vi "forwardByNavX_theSide(queuesWithNavX).vi"(8 "error in (no error)":errorcluster, 11 "distance the side":u32) -> (0 "error out":errorcluster)   [LabVIEW 2017]
uses:
  <vilib>/myRIO/Common/Instrument Driver Framework/Utilities/typedefs/FPGA Ref Manager Action Enum.ctl
  <vilib>/myRIO/Instrument Drivers/Onboard IO/I2C/typedefs/I2C Reference.ctl
  <vilib>/myRIO/Common/Instrument Driver Framework/Utilities/typedefs/myRIO Generic Hardware Reference.ctl
  <vilib>/myRIO/Common/Instrument Driver Framework/Utilities/typedefs/Hardware Version Enum.ctl
  <vilib>/myRIO/Common/Instrument Driver Framework/Utilities/typedefs/myRIO v1.0 Reference.ctl
  <vilib>/myRIO/Common/Instrument Driver Framework/Utilities/typedefs/Generic FPGA Reference.ctl
  <vilib>/myRIO/Common/Instrument Driver Framework/myRIO v1.0/I2C/typedefs/I2C Channels Enum.ctl
  <vilib>/myRIO/Instrument Drivers/Onboard IO/I2C/typedefs/I2C Configuration.ctl
  <vilib>/myRIO/Instrument Drivers/Onboard IO/I2C/typedefs/I2C Transfer Rate.ctl
  <vilib>/userdefined/High Color/nirio_resource_hc.ctl
  <vilib>/myRIO/Common/Instrument Driver Framework/myRIO v1.0/I2C/vis/myRIO v1.1 Open I2C.vi
  <vilib>/myRIO/Common/Instrument Driver Framework/Utilities/vis/Validate Channels.vi
  <vilib>/myRIO/Common/Instrument Driver Framework/myRIO v1.0/I2C/vis/myRIO v1.0 Reserve I2C.vi
  <vilib>/myRIO/Common/Instrument Driver Framework/myRIO v1.0/I2C/vis/myRIO v1.0 Close I2C.vi
  <vilib>/myRIO/Common/Instrument Driver Framework/myRIO v1.0/I2C/vis/myRIO v1.0 Build MUX Configuration I2C.vi
  <vilib>/myRIO/Common/Instrument Driver Framework/myRIO v1.0/Resource Manager/vis/myRIO v1.0 Reserve Channel List.vi
  <vilib>/myRIO/Common/Instrument Driver Framework/myRIO v1.0/I2C/vis/myRIO v1.0 Unreserve I2C.vi
  <vilib>/myRIO/Common/Instrument Driver Framework/myRIO v1.0/Resource Manager/vis/myRIO v1.0 Create Configuration List.vi
  <vilib>/myRIO/Common/Instrument Driver Framework/myRIO v1.0/Resource Manager/vis/myRIO v1.0 Reserve Channel.vi
  <vilib>/myRIO/Common/Instrument Driver Framework/myRIO v1.0/Resource Manager/vis/myRIO v1.0 Unreserve Channel.vi
  <vilib>/myRIO/Common/Instrument Driver Framework/myRIO v1.0/Resource Manager/vis/myRIO v1.0 Unreserve Channel List.vi
  <vilib>/myRIO/Common/Instrument Driver Framework/myRIO v1.0/Resource Manager/vis/myRIO v1.0 Build Mutex Name.vi
  <vilib>/Utility/VariantDataType/GetNumericInfo.vi
  <vilib>/Utility/error.llb/Error Cluster From Error Code.vi
  <vilib>/myRIO/Common/Instrument Driver Framework/myRIO v1.0/myRIO v1.1 Open.vi
  <vilib>/myRIO/Common/Instrument Driver Framework/Utilities/vis/IO Manager.vi
  <vilib>/myRIO/Common/Instrument Driver Framework/Utilities/vis/Configuration Manager.vi
  <vilib>/myRIO/Common/Instrument Driver Framework/myRIO v1.0/Resource Manager/vis/myRIO v1.0 Configure IO.vi
  <vilib>/myRIO/Common/Instrument Driver Framework/myRIO v1.0/myRIO v1.0 Close.vi
  <vilib>/Instr/_visa.llb/VISA Configure Serial Port (Instr).vi
  <vilib>/myRIO/Common/Instrument Driver Framework/myRIO v1.0/I2C/vis/myRIO v1.0 Shutdown I2C.vi
  <vilib>/myRIO/Instrument Drivers/Onboard IO/I2C/vis/myRIO I2C Open.xnode
  <vilib>/myRIO/Instrument Drivers/Onboard IO/I2C/I2C.lvlib
panel:
  out "axis Z(paste)":ext
  out "main angle":ext
  out "right":dbl
  out "left":dbl
  out "zero angle":ext
  in  "Stop Button":bool
  out "axis Z(after)":ext
  # "--- отклонения от нулевого угла"
  # "PWM"
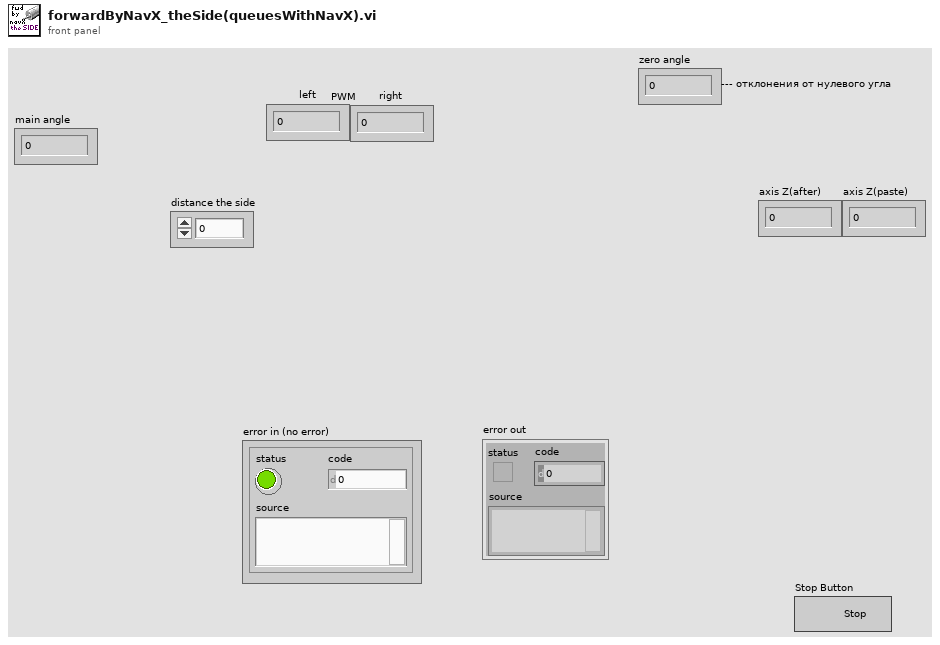
[diagram p1: front panel]
types:
  T1 = typedef "FPGA Ref Manager Action Enum.ctl" = enum16{"Get", "Set", "Reset"}
  T2 = typedef "I2C.lvlib/I2C Reference.ctl" = cluster{"myRIO Reference":T3, "I2C Channels Enum":T7, "I2C Configuration":T8}
  T3 = typedef "myRIO Generic Hardware Reference.ctl" = cluster{"myRIO Model":T4, "myRIO Hardware Reference":T5}
  T4 = typedef "Hardware Version Enum.ctl" = enum16{"Unknown", "myRIO-1900", "myRIO-1950", "roboRIO", "NI ELVIS RIO CM"}
  T5 = typedef "myRIO v1.0 Reference.ctl" = cluster{"Generic FPGA Reference":T6, "Allow multiple opens":bool}
  T6 = typedef "Generic FPGA Reference.ctl" = refnum<k20>
  T7 = typedef "I2C Channels Enum.ctl" = enum16{"Not Connected", "A/I2C", "B/I2C", "I2C/I2C"}
  T8 = typedef "I2C.lvlib/I2C Configuration.ctl" = cluster{"I2C Transfer Rate":T9}
  T9 = typedef "I2C.lvlib/I2C Transfer Rate.ctl" = enum16{"Standard mode (100 kbps)", "Fast mode (400 kbps)"}
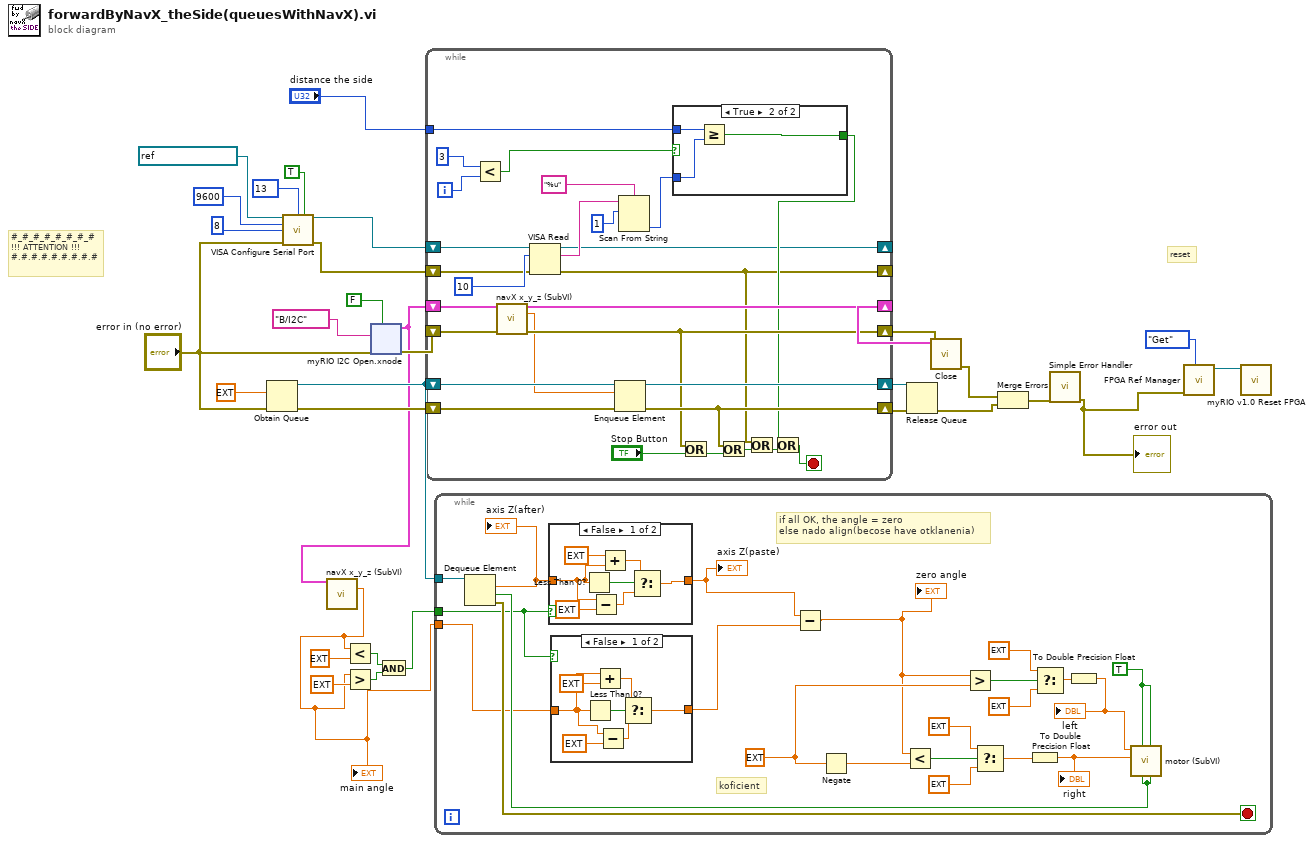
[diagram p0: block diagram]
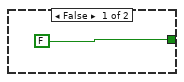
[diagram p4: hidden frame]
diagram:
  # "#_#_#_#_#_#_#_#\n!!! ATTENTION !!!\n#.#.#.#.#.#.#.#.#"
  # "reset"
  n1 = Obtain Queue(element data type=ext 0.0 ("value Z"), error in (no error)="error in (no error)") -> (queue out=w20:refnum<queue>, error out=w32:errorcluster)  [unwired: 3 in, 1 out]
  n2 = call-poly "VISA Configure Serial Port"("VISA resource name"=refnum<visa-resource-name> "ASRL2::INSTR" ("UART selector"), "termination char\n(0xA = '\\n' = LF)"=u8 13 ("termination char = CR"), "Enable Termination\nChar (T)"=TRUE ("enable termination char"), "baud rate (9600)"=u32 9600 ("baud rate"), "data bits (8)"=u16 8 ("data bits"), "error in (no error)"="error in (no error)") -> ("VISA resource name out"=w2:refnum<visa-resource-name>, "error out"=w3:errorcluster)  [unwired: 8 in]
  n3 = xnode "myRIO I2C Open.xnode"("error in (no error)"="error in (no error)", "Allow multiple opens?"=FALSE, "Channel Name"=tag "B/I2C") -> ("error out"=w25:errorcluster, "I2C Ref Out"=w16:T2)
  n4 = call "navX x_y_z (SubVI).vi"("I2C Ref Out in"=w16) -> ("value Z"=w13:ext)  [unwired: 10 in, 4 out]
  "main angle" <- w13
  n5 = Less?(x=w13, y=ext 90.0) -> (x < y?=w11:bool)
  n6 = Greater?(x=w13, y=ext -90.0) -> (0:w14:bool)
  n7 = And(x=w11, y=w14) -> (x .and. y?=w10:bool)
  n8 = while {
    shift-right: [w54] -> w30
    shift-left: w32 -> [w59]
    shift-right: [w58] -> w31
    shift-left: w20 -> [w60]
    shift-right: [w55] -> w26
    shift-left: w16 -> [w56]
    shift-right: [w51] -> w24
    shift-left: w25 -> [w52]
    tunnel: "distance the side" -> [w38]
    shift-right: [w33] -> _
    shift-left: w3 -> [w40]
    shift-right: [w35] -> _
    shift-left: w2 -> [w39]
    i -> [w37]
    stop <- w48 stop-if-true
    n9 = Less?(x=3, y=w37) -> (x < y?=w41:bool)
    n10 = call "navX x_y_z (SubVI).vi"("I2C Ref Out in"=w56, "error in (no error)"=w52) -> ("I2C Ref Out out"=w55:T2, "value Z"=w50:ext, "error out"=w51:errorcluster)  [unwired: 9 in, 2 out]
    n11 = VISA Read(VISA resource name=w39, byte count=u32 10, error in (no error)=w40) -> (VISA resource name out=w35:refnum<visa-resource-name>, read buffer=w44:string, error out=w33:errorcluster)  [unwired: 1 out]
    n12 = Enqueue Element(queue=w60, element=w50, error in (no error)=w59) -> (queue out=w58:refnum<queue>, error out=w54:errorcluster)  [unwired: 1 in, 1 out]
    n13 = Scan From String(format string="%u", input string=w44, initial scan location=u32 1) -> (output 1=w43:u32)  [unwired: 2 in, 3 out]
    n14 = case shown="True" w41 {
      tunnel: w43 -> [_ w64]
      tunnel: w38 -> [_ w63]
      tunnel: [FALSE w62] -> w36
      frame False {
      }
      frame True {
        n15 = Greater Or Equal?(x=w63, y=w64) -> (x >= y?=w62:bool)
      }
    }
    n16 = Or(x=w51, y="Stop Button") -> (x .or. y?=w53:bool)
    n17 = Or(x=w54, y=w53) -> (x .or. y?=w49:bool)
    n18 = Or(x=w33, y=w49) -> (x .or. y?=w34:bool)
    n19 = Or(x=w36, y=w34) -> (x .or. y?=w48:bool)
  }
  n20 = while {
    tunnel: w20 -> [w86]
    tunnel: w13 -> [w68]
    tunnel: w10 -> [w67]
    stop <- w85 stop-if-true
    w74 = TRUE ("M0 (Pin 21)")
    w78 = ext 1.0 ("y")
    # "koficient"
    # "if all OK, the angle = zero\nelse nado align(becose have otklanenia)"
    n21 = Dequeue Element(queue=w86) -> (element=w70:ext, timed out?=w73:bool, error out=w85:errorcluster)  [unwired: 2 in, 1 out]
    "axis Z(after)" <- w70
    n22 = case shown="False" w67 {
      tunnel: [w100 w102] -> w71
      tunnel: w70 -> [w96 w102]
      frame False {
        n23 = Less Than 0?(x=w96) -> (x < 0?=w101:bool)
        n24 = Subtract(x=w96, y=ext 180.0) -> (x-y=w97:ext)
        n25 = Add(x=ext 180.0, y=w96) -> (x+y=w99:ext)
        n26 = Select(t=w99, s=w101, f=w97) -> (s? t:f=w100:ext)
      }
      frame True {
      }
    }
    "axis Z(paste)" <- w71
    n27 = case shown="False" w67 {
      tunnel: [w92 w94] -> w69
      tunnel: w68 -> [w89 w94]
      frame False {
        n28 = Less Than 0?(x=w89) -> (x < 0?=w93:bool)
        n29 = Add(x=w89, y=ext 180.0) -> (x+y=w91:ext)
        n30 = Subtract(x=w89, y=ext 180.0) -> (x-y=w90:ext)
        n31 = Select(t=w91, s=w93, f=w90) -> (s? t:f=w92:ext)
      }
      frame True {
      }
    }
    n32 = Subtract(x=w71, y=w69) -> (x-y=w72:ext)
    "zero angle" <- w72
    n33 = Negate(x=w78) -> (-x=w77:ext)
    n34 = Less?(x=w72, y=w77) -> (x < y?=w81:bool)
    n35 = Greater?(x=w72, y=w78) -> (0:w84:bool)
    n36 = Select(t=ext 0.2 ("y"), s=w81, f=ext 0.4 ("y")) -> (s? t:f=w75:ext)
    n37 = To Double Precision Float(number=w75) -> (double precision float=w66:dbl)
    "right" <- w66
    n38 = Select(t=ext 0.2 ("y"), s=w84, f=ext 0.4 ("y")) -> (s? t:f=w76:ext)
    n39 = To Double Precision Float(number=w76) -> (double precision float=w65:dbl)
    "left" <- w65
    n40 = call "motor (SubVI).vi"("M1 (Pin 26)"=w73, "M1 (Pin 25)"=w74, "M0 (Pin 23)"=w73, "M0 (Pin 21)"=w74, "PWM1"=w66, "PWM0"=w65) -> ()  [unwired: 5 in, 1 out]
  }
  n41 = Release Queue(queue=w31, error in (no error)=w30) -> (error out=w21:errorcluster)  [unwired: 1 in, 2 out]
  n42 = call <vilib>:"Close.vi"("error in (no error)"=w24, "I2C Ref In"=w26) -> ("error out"=w22:errorcluster)  [unwired: 9 in]
  n43 = Merge Errors(w22, w21) -> (w23:errorcluster)
  n44 = call <vilib>:"Simple Error Handler.vi"("error in (no error)"=w23) -> ("error out"=w17:errorcluster)  [unwired: 4 in, 4 out]
  "error out" <- w17
  n45 = call <vilib>:"FPGA Ref Manager.vi"("Action"=FPGA_Ref_Manager_Action_Enum."Get" ("Ref Counter Action Enum"), "error in (no error)"=w17) -> ("Generic FPGA Reference out"=w19:T6)  [unwired: 7 in, 1 out]
  n46 = call <vilib>:"myRIO v1.0 Reset FPGA.vi"("Generic FPGA Reference in"=w19) -> ()  [unwired: 9 in, 2 out]
